vi "MC_DAQ_thermocouple_BM_subVI.vi"(8 "BitNum":u32=1, 11 "BoardNum":u32) -> (0 "Error code":i32, 3 "Temp (oC)":dbl=23.199816942214966 format="%_6g")   [LabVIEW 2021]
uses:
  <vilib>/ULx/Create Channel.llb/ULx Create Channel (AI-Voltage-Basic).vi
  <vilib>/ULx/Read.llb/ULx Read (Analog DBL 1Chan 1Samp).vi
panel:
  out "Raw Voltage":dbl=0.09666590392589569 format="%_6g"
  in  "min V":dbl=-5.0
  in  "max V":dbl=5.0
  out "error out":errorcluster
  in  "error in":errorcluster
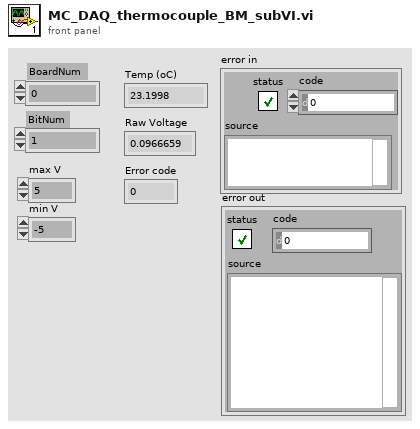
[diagram p1: front panel]
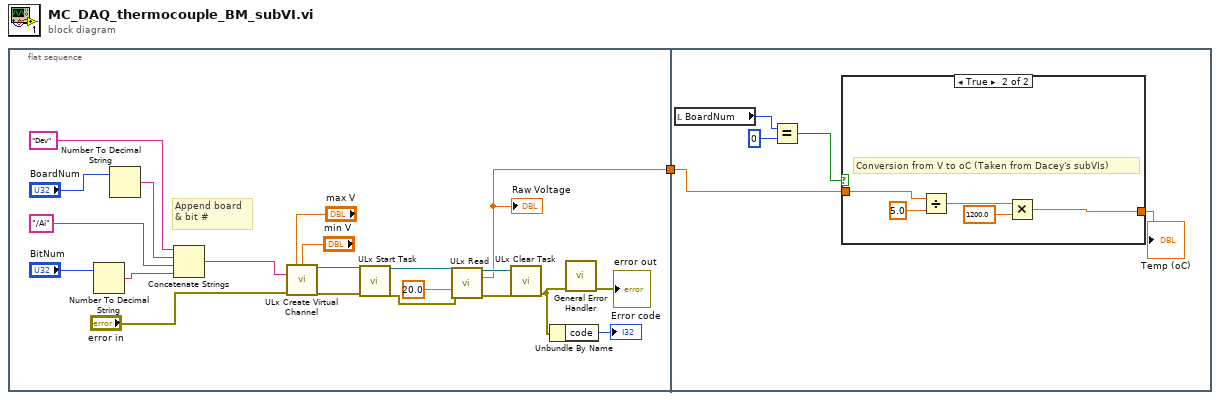
[diagram p0: block diagram]
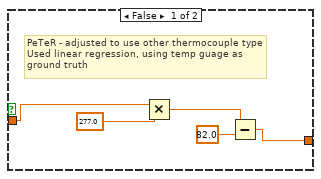
[diagram p2: hidden frame]
diagram:
  n1 = flat-sequence {
    tunnel: [w11] -> w1
    tunnel: w1 -> [w23]
    frame #0 {
      # "Append board\n& bit #"
      n2 = Number To Decimal String(number="BitNum") -> (decimal integer string=w17:string)  [unwired: 1 in]
      n3 = Number To Decimal String(number="BoardNum") -> (decimal integer string=w16:string)  [unwired: 1 in]
      n4 = Concatenate Strings("Dev", w16, "/Ai", w17) -> (w14:string)
      n5 = call-poly <vilib>:"ULx Create Virtual Channel.vi"("maximum value"="max V", "minimum value"="min V", "physical channels"=w14, "error in"="error in") -> ("task out"=w7:refnum<k24>, "error out"=w4:errorcluster)  [unwired: 10 in]
      n6 = call <vilib>:"ULx Start Task.vi"("task in"=w7, "error in"=w4) -> ("task out"=w6:refnum<k24>, "error out"=w5:errorcluster)  [unwired: 12 in]
      n7 = call-poly <vilib>:"ULx Read.vi"("task in"=w6, "timeout"=20.0, "error in"=w5) -> ("task out"=w22:refnum<k24>, "data"=w11:dbl, "error out"=w20:errorcluster)  [unwired: 10 in]
      "Raw Voltage" <- w11
      n8 = call <vilib>:"ULx Clear Task.vi"("task in"=w22, "error in"=w20) -> ("error out"=w3:errorcluster)  [unwired: 13 in]
      n9 = Unbundle By Name(w3) -> ("code"=→"Error code":i32)
      n10 = call <vilib>:"General Error Handler.vi"("error in (no error)"=w3) -> ("error out"=→"error out":errorcluster)  [unwired: 10 in, 4 out]
    }
    frame #1 {
      n11 = local read "BoardNum"() -> (w27:u32)
      n12 = Equal?(x=w27, y=u32 0) -> (x = y?=w26:bool)
      n13 = case shown="True" w26 {
        tunnel: [w29 w34] -> w24
        tunnel: w23 -> [w28 w33]
        frame False {
          # "PeTeR - adjusted to use other thermocouple type\nUsed linear regression, using temp guage as ground truth"
          n14 = Multiply(x=w28, y=277.0) -> (x*y=w31:dbl)
          n15 = Subtract(x=w31, y=82.0) -> (x-y=w29:dbl)
        }
        frame True {
          # "Conversion from V to oC (Taken from Dacey's subVIs)"
          n16 = Divide(x=w33, y=5.0) -> (x/y=w36:dbl)
          n17 = Multiply(x=w36, y=1200.0) -> (x*y=w34:dbl)
        }
      }
      "Temp (oC)" <- w24
    }
  }
